vi "Load Scripting Controls Panel.vi"(11 "SubPanel in":refnum<vi>) -> ()   [LabVIEW 2019, in "Panther Dashboard.lvlib"]
uses:
  Panther Dashboard.lvlib
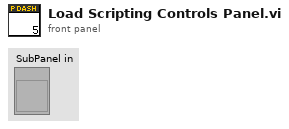
[diagram p1: front panel]
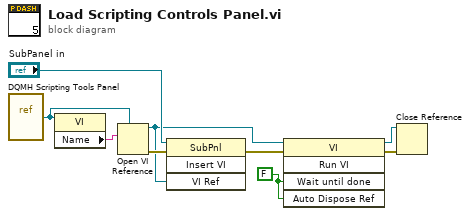
[diagram p0: block diagram]
diagram:
  w2 = FALSE ("Wait Until Done")
  n1 = vi-ref "DQMH Scripting Tools Panel.vi"() -> (w9:refnum<vi>)
  n2 = property class="VI"(reference=w9) -> ("Name"=w8:string)  [unwired: 1 in, 2 out]
  n3 = Open VI Reference(type specifier VI Refnum (for type only)=w9, vi path=w8) -> (vi reference=w1:refnum<vi>, error out=w5:errorcluster)  [unwired: 4 in]
  n4 = invoke class="SubPnl" method="Insert VI"(reference="SubPanel in", error in=w5, "VI Ref"=w1) -> (error out=w6:errorcluster)  [unwired: 1 in, 3 out]
  n5 = invoke class="VI" method="Run VI"(reference=w1, error in=w6, "Wait until done"=w2, "Auto Dispose Ref"=w2) -> (reference out=w3:refnum<vi>, error out=w4:errorcluster)  [unwired: 1 in, 3 out]
  n6 = Close Reference(reference=w3, error in (no error)=w4) -> ()  [unwired: 1 out]
